vi "C - F temp conversion.vi"() -> ()   [LabVIEW 2018]
panel:
  in  "Boolean":bool
  out "Temp C":dbl
  out "Temp F":dbl
  out "Temp C":dbl(slide) scale=0.0..200.0
  in  "Temp F":dbl(slide) scale=0.0..200.0
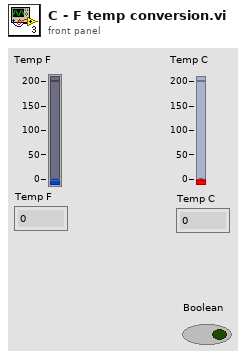
[diagram p1: front panel]
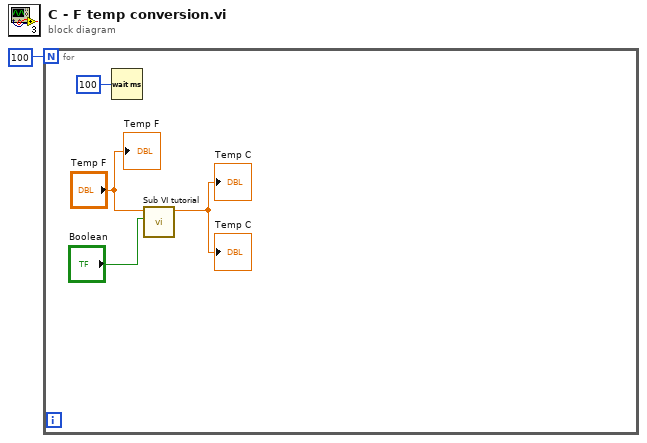
[diagram p0: block diagram]
diagram:
  n1 = for {
    N: 100 -> [_]
    n2 = Wait (ms)(milliseconds to wait=100) -> ()  [unwired: 1 out]
    n3 = call "Sub VI tutorial.vi"("Boolean"="Boolean", "Temp F"="Temp F") -> ("Numeric"=→"Temp C" →"Temp C":dbl)  [unwired: 9 in]
    "Temp F" <- "Temp F"
  }
